vi "winForms initConfiguration.vi"(4 "editorType":T1, 6 "initText":string, 8 "error in (no error)":errorcluster, 10 "scintillaRefNum in":refnum<k24>, 11 "panelRefNum":refnum<k24>) -> (0 "error out":errorcluster, 2 "scintillaRefNum out":refnum<k24>)   [LabVIEW 2018]
uses:
  C:/ATI_MS_InstrumentControl/dll/ScintillaNET.dll
  dll/ScintillaNET.dll
  System.Windows.Forms
  winForms editorType.ctl
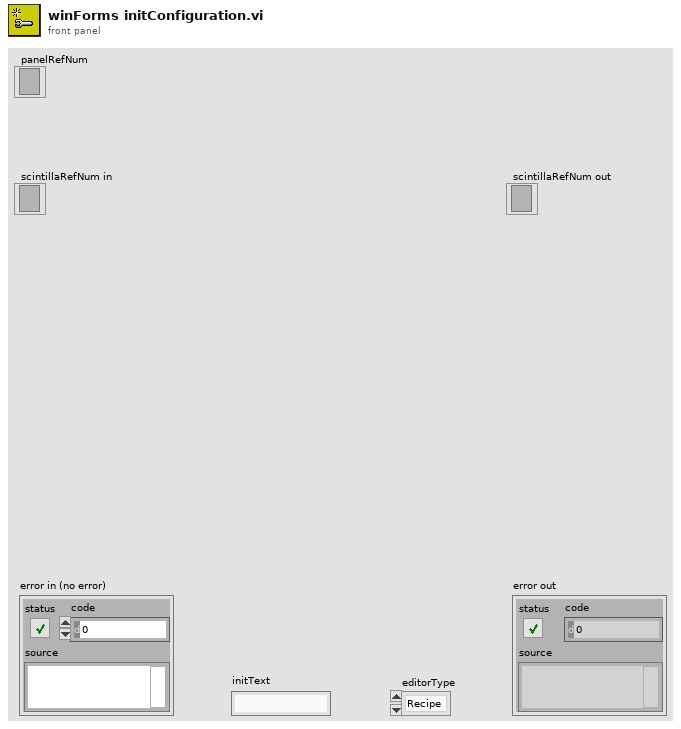
[diagram p1: front panel]
types:
  T1 = typedef "winForms editorType.ctl" = enum16{"Recipe", "SigProc", "Editor"}
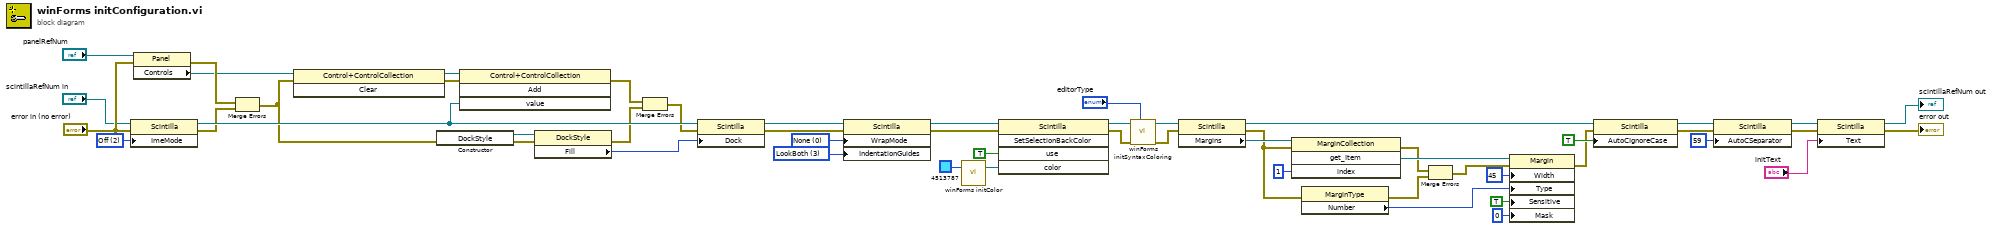
[diagram p0: block diagram]
diagram:
  w39 = 3 items=["None", "Real", "LookForward", "LookBoth"] ("IndentationGuides")
  w40 = 0 items=["None", "Word", "Char", "Whitespace"] ("WrapMode")
  w50 = 2 items=["NoControl"=0, "On"=1, "Off"=2, "Disable"=3, "Hiragana"=4, "Katakana"=5, "KatakanaHalf"=6, "AlphaFull"=7, "Alpha"=8, "HangulFull"=9, "Hangul"=10, "Close"=11, "OnHalf"=12, "Inherit"=-1] ("ImeMode")
  n1 = property class="Scintilla"(reference="scintillaRefNum in", error in="error in (no error)", "ImeMode"=w50) -> (reference out=w49:refnum<k24>, error out=w44:errorcluster)
  n2 = property class="Panel"(reference="panelRefNum", error in="error in (no error)") -> (error out=w45:errorcluster, "Controls"=w10:refnum<k24>)  [unwired: 1 out]
  n3 = Merge Errors(w45, w44) -> (w7:errorcluster)
  n4 = invoke class="Control+ControlCollection" method="Clear"(reference=w10, error in=w7) -> (reference out=w9:refnum<k24>, error out=w8:errorcluster)  [unwired: 1 in, 1 out]
  n5 = constructor class="DockStyle"(error in=w7) -> (reference out=w53:refnum<k24>, error out=w52:errorcluster)  [unwired: 2 in, 1 out]
  n6 = invoke class="Control+ControlCollection" method="Add"(reference=w9, error in=w8, "value"=w49) -> (error out=w42:errorcluster)  [unwired: 1 in, 3 out]
  n7 = property class="DockStyle"(reference=w53, error in=w52) -> (error out=w43:errorcluster, "Fill"=w51:i32)  [unwired: 1 out]
  n8 = Merge Errors(w42, w43) -> (w41:errorcluster)
  n9 = property class="Scintilla"(reference=w49, error in=w41, "Dock"=w51) -> (reference out=w33:refnum<k24>, error out=w32:errorcluster)
  n10 = property class="Scintilla"(reference=w33, error in=w32, "WrapMode"=w40, "IndentationGuides"=w39) -> (reference out=w35:refnum<k24>, error out=w34:errorcluster)
  n11 = call "winForms initColor.vi"("Color Box"=u32 4513787) -> ("reference out"=w36:refnum<k24>)  [unwired: 1 in, 1 out]
  n12 = invoke class="Scintilla" method="SetSelectionBackColor"(reference=w35, error in=w34, "use"=TRUE, "color"=w36) -> (reference out=w31:refnum<k24>, error out=w30:errorcluster)  [unwired: 1 in, 3 out]
  n13 = call "winForms initSyntaxColoring.vi"("editorType"="editorType", "error in (no error)"=w30, "scintillaRefNum in"=w31) -> ("error out"=w28:errorcluster, "scintillaRefNum out"=w29:refnum<k24>)  [unwired: 5 in]
  n14 = property class="Scintilla"(reference=w29, error in=w28) -> (reference out=w12:refnum<k24>, error out=w20:errorcluster, "Margins"=w21:refnum<k24>)
  n15 = invoke class="MarginCollection" method="get_Item"(reference=w21, error in=w20, "index"=1) -> (error out=w18:errorcluster, "get_Item"=w26:refnum<k24>)  [unwired: 1 in, 2 out]
  n16 = property class="MarginType"(error in=w20) -> (error out=w19:errorcluster, "Number"=w24:i32)  [unwired: 1 in, 1 out]
  n17 = Merge Errors(w18, w19) -> (w17:errorcluster)
  n18 = property class="Margin"(reference=w26, error in=w17, "Width"=45, "Type"=w24, "Sensitive"=TRUE, "Mask"=u32 0) -> (error out=w11:errorcluster)  [unwired: 1 out]
  n19 = property class="Scintilla"(reference=w12, error in=w11, "AutoCIgnoreCase"=TRUE) -> (reference out=w14:refnum<k24>, error out=w13:errorcluster)
  n20 = property class="Scintilla"(reference=w14, error in=w13, "AutoCSeparator"=u16 59) -> (reference out=w5:refnum<k24>, error out=w4:errorcluster)
  n21 = property class="Scintilla"(reference=w5, error in=w4, "Text"="initText") -> (reference out=→"scintillaRefNum out":refnum<k24>, error out=→"error out":errorcluster)
